vi "Tab Page Toggle.vi"() -> ()   [LabVIEW 2022 SP3]
panel:
  in  "OK Button 3":bool
  in  "stop":bool
  in  "OK Button 2":bool
  in  "OK Button":bool
  in  "Tab Control":enum32{"Page 1", "Page 3", "Page 2"}(tab)
  out "Gauge":dbl(knob) scale=0.0..10.0
  out "Meter":dbl(knob) scale=0.0..10.0
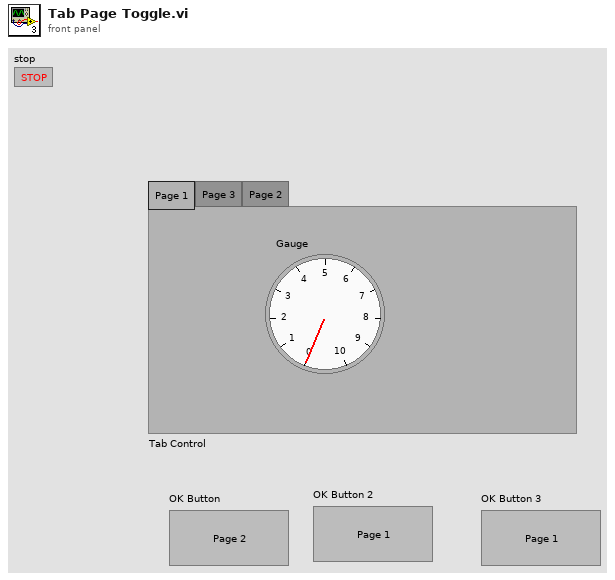
[diagram p1: front panel]
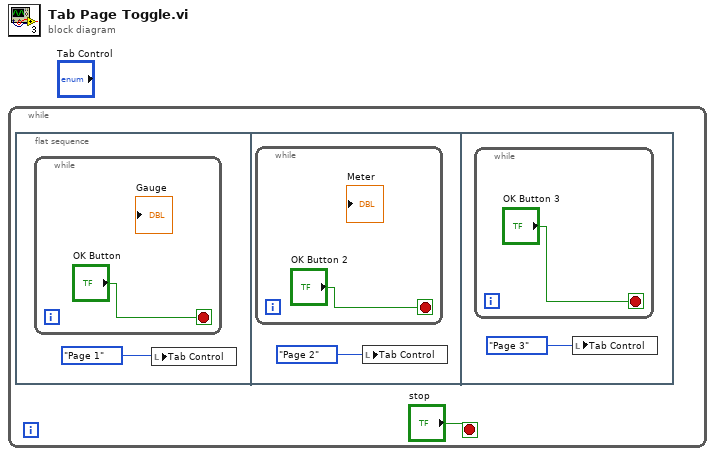
[diagram p0: block diagram]
diagram:
  n1 = while {
    stop <- "stop" stop-if-true
    n2 = flat-sequence {
      frame #0 {
        n3 = while {
          stop <- "OK Button" stop-if-true
        }
        n4 = local write "Tab Control"(enum32{"Page 1", "Page 3", "Page 2"}."Page 1" ("Tab Control")) -> ()
      }
      frame #1 {
        n5 = while {
          stop <- "OK Button 2" stop-if-true
        }
        n6 = local write "Tab Control"(enum32{"Page 1", "Page 3", "Page 2"}."Page 2" ("Tab Control")) -> ()
      }
      frame #2 {
        n7 = while {
          stop <- "OK Button 3" stop-if-true
        }
        n8 = local write "Tab Control"(enum32{"Page 1", "Page 3", "Page 2"}."Page 3" ("Tab Control")) -> ()
      }
    }
  }
